vi "19052_Get_STATUS.vi"(8 "error in (no error)":errorcluster, 11 "VISA resource in":refnum<visa-resource-name>) -> (0 "error out":errorcluster, 1 "Status":string, 3 "VISA resource out":refnum<visa-resource-name>)   [LabVIEW 2015]
panel:
  out "output command":string
  # "Get STATUS"
  # "This is valid for both:\n19572 & 19052"
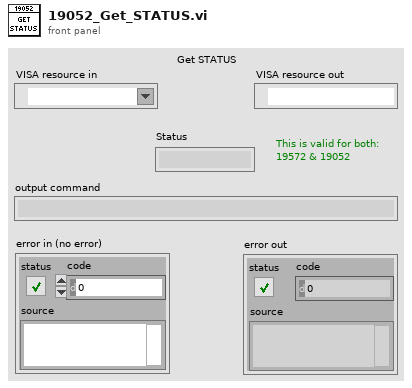
[diagram p1: front panel]
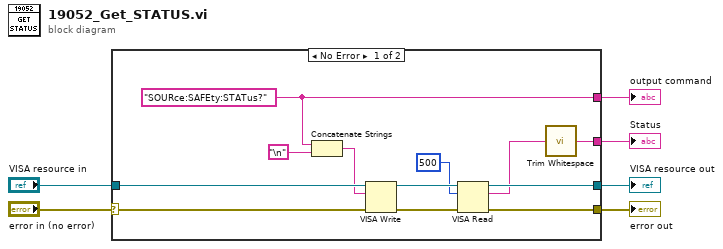
[diagram p0: block diagram]
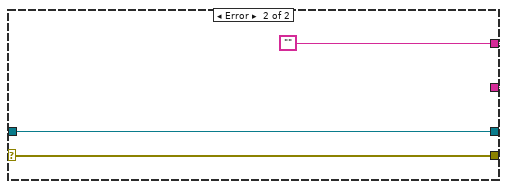
[diagram p2: hidden frame]
diagram:
  n1 = case shown="No Error" "error in (no error)" {
    selector: "error in (no error)" -> [w13 w21]
    tunnel: [w18 w21] -> w6
    tunnel: "VISA resource in" -> [w17 w20]
    tunnel: [w12 w19] -> w4
    tunnel: [w14 w20] -> w3
    tunnel: [w10 w19] -> w2
    frame No Error {
      w12 = "SOURce:SAFEty:STATus?"
      n2 = Concatenate Strings(w12, "\n") -> (w15:string)
      n3 = VISA Write(VISA resource name=w17, write buffer=w15, error in (no error)=w13) -> (VISA resource name out=w9:refnum<visa-resource-name>, error out=w8:errorcluster)  [unwired: 1 out]
      n4 = VISA Read(VISA resource name=w9, byte count=u32 500, error in (no error)=w8) -> (VISA resource name out=w14:refnum<visa-resource-name>, read buffer=w11:string, error out=w18:errorcluster)  [unwired: 1 out]
      n5 = call <vilib>:"Trim Whitespace.vi"("string"=w11) -> ("trimmed string"=w10:string)  [unwired: 1 in]
    }
    frame Error {
      w19 = ""
    }
  }
  "error out" <- w6
  "VISA resource out" <- w3
  "output command" <- w4
  "Status" <- w2
